vi "IntervalTime.vi"(9 "Cluster out":T2, 11 "output cluster":T1) -> (1 "close":bool, 3 "output cluster 2":T1)   [LabVIEW 2013]
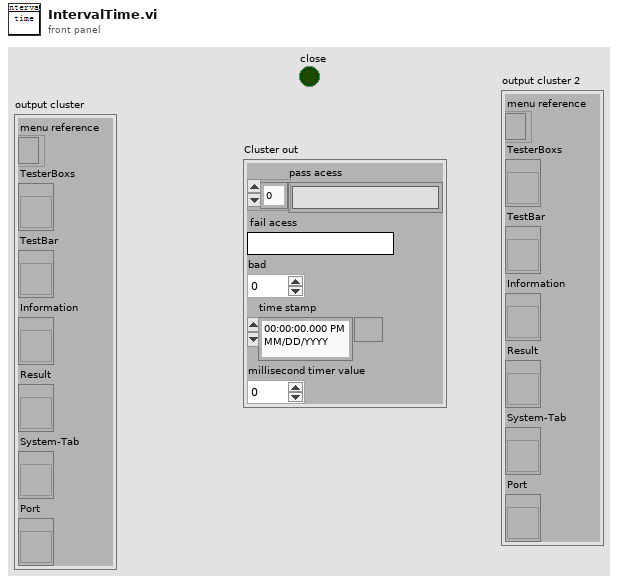
[diagram p1: front panel]
types:
  T1 = cluster{"menu reference":refnum<k9>, "TesterBoxs":refnum<vi>, "TestBar":refnum<vi>, "Information":refnum<vi>, "Result":refnum<vi>, "System-Tab":refnum<vi>, "Port":refnum<vi>}
  T2 = cluster{"pass acess":string[], "fail acess":string, "bad":i32, "time stamp":timestamp, "millisecond timer value":u32}
  T3 = typedef "StatusInformation.ctl" = cluster{"FileName:":string, "Barcode(S/N):":string, "TestStep:":string, "TestTime:":string, "Station:":string, "Model:":string, "Line:":string, "Status:":string, "Series:":string, "Reserve:":string}
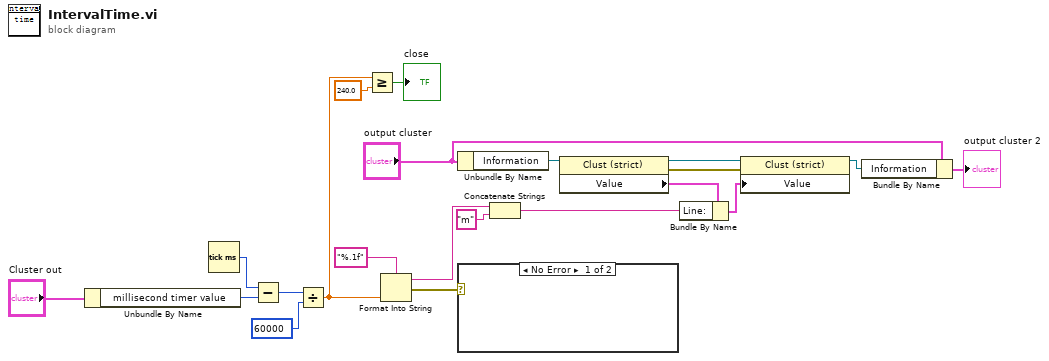
[diagram p0: block diagram]
diagram:
  n1 = Unbundle By Name("Cluster out") -> ("millisecond timer value"=w19:u32)
  n2 = Tick Count (ms)() -> (millisecond timer value=w21:u32)
  n3 = Subtract(x=w21, y=w19) -> (x-y=w18:u32)
  n4 = Divide(x=w18, y=u32 60000) -> (x/y=w6:dbl)
  n5 = Greater Or Equal?(x=w6, y=240.0) -> (x >= y?=→"close":bool)
  n6 = Format Into String(format string="%.1f", w6) -> (resulting string=w3:string, error out=w15:errorcluster)  [unwired: 2 in]
  n7 = Unbundle By Name("output cluster") -> ("Information"=w14:refnum<vi>)
  n8 = case shown="No Error" w15 {
    frame No Error {
    }
    frame Error {
    }
  }
  n9 = Concatenate Strings(w3, "m" ("string")) -> (w1:string)
  n10 = property class="Clust (strict)"(reference=w14) -> (reference out=w12:refnum<vi>, error out=w11:errorcluster, "Value"=w13:T3)  [unwired: 1 in]
  n11 = Bundle By Name(cluster=w13, "Line:"=w1) -> (w10:T3)
  n12 = property class="Clust (strict)"(reference=w12, error in=w11, "Value"=w10) -> (reference out=w8:refnum<vi>)  [unwired: 1 out]
  n13 = Bundle By Name(cluster="output cluster", "Information"=w8) -> (→"output cluster 2":T1)
